vi "test_client_builder_configured.vi"() -> ()   [LabVIEW 2020, in "reqwest_tests.lvlib"]
uses:
  reqwest_tests.lvlib
  <vilib>/addons/_JKI Toolkits/Caraya/classes/Assert/Assert.lvclass
  <vilib>/addons/_JKI Toolkits/Caraya/classes/Test/Test.lvclass
  ClientBuilder/ClientBuilder.lvclass
  Client/Client.lvclass
panel:
  in  "error in (no error)":errorcluster
  out "error out":errorcluster
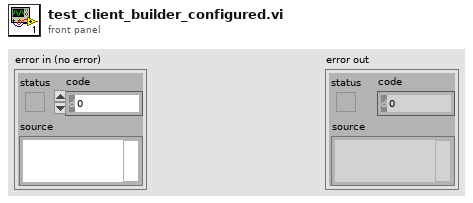
[diagram p1: front panel]
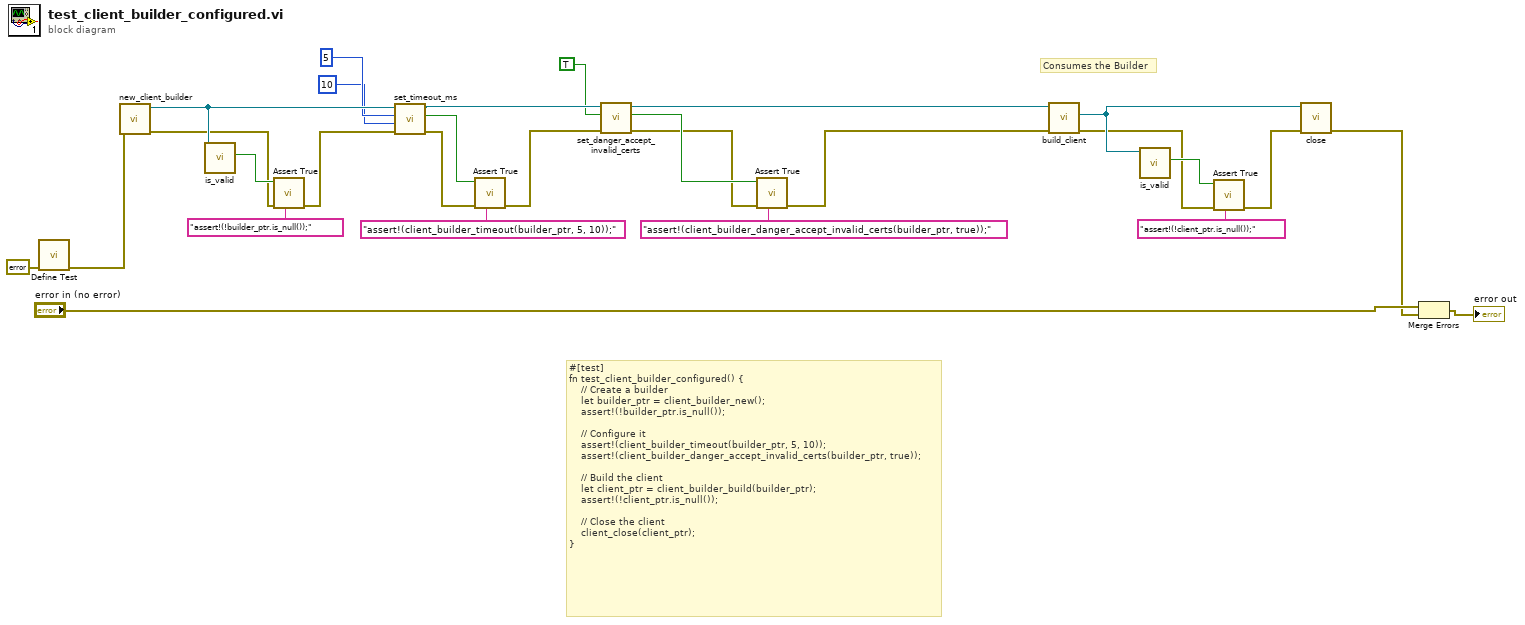
[diagram p0: block diagram]
diagram:
  # "Consumes the Builder"
  # "#[test]\nfn test_client_builder_configured() {\n    // Create a builder\n    let builder_ptr = client_builder_new();\n    assert!(!builder_ptr.is_null());\n\n    // Configure it\n    assert!(client_builder_timeout(builder_ptr, 5, 10));\n    assert!(client_builder_danger_accept_invalid_certs(builder_ptr, true));\n\n    // Build the client\n    let client_ptr = client_builder_build(builder_ptr);\n    assert!(!client_ptr.is_null());\n\n    // Close the client\n    client_close(client_ptr);\n}"
  n1 = call <vilib>:"Define Test.vi"("error in (no error)"=errorcluster {"status"=FALSE, "code"=0, "source"=""}) -> ("error out"=w9:errorcluster)  [unwired: 9 in, 1 out]
  n2 = call "new_client_builder.vi"("error in (no error)"=w9) -> ("error out"=w8:errorcluster, "Client out"=w23:refnum<class "ClientBuilder.lvclass">)  [unwired: 9 in]
  n3 = call "is_valid.vi"("Client in"=w23) -> ("valid-ref?"=w25:bool)  [unwired: 10 in]
  n4 = call <vilib>:"Assert True.vi"("Label"="assert!(!builder_ptr.is_null());", "error in (no error)"=w8, "True?"=w25) -> ("error out"=w7:errorcluster)  [unwired: 7 in, 1 out]
  n5 = call "set_timeout_ms.vi"("error in (no error)"=w7, "timeout_secs"=u64 10, 10:u64 5 ("connect_timeout_secs"), "ClientBuilder in"=w23) -> ("error out"=w6:errorcluster, "success"=w19:bool, "ClientBuilder out"=w18:refnum<class "ClientBuilder.lvclass">)  [unwired: 5 in]
  n6 = call <vilib>:"Assert True.vi"("Label"="assert!(client_builder_timeout(builder_ptr, 5, 10));", "error in (no error)"=w6, "True?"=w19) -> ("error out"=w5:errorcluster)  [unwired: 7 in, 1 out]
  n7 = call "set_danger_accept_invalid_certs.vi"("error in (no error)"=w5, "danger_accept_invalid_certs"=TRUE, "ClientBuilder in"=w18) -> ("error out"=w4:errorcluster, "success"=w15:bool, "ClientBuilder out"=w14:refnum<class "ClientBuilder.lvclass">)  [unwired: 6 in]
  n8 = call <vilib>:"Assert True.vi"("Label"="assert!(client_builder_danger_accept_invalid_certs(builder_ptr, true));", "error in (no error)"=w4, "True?"=w15) -> ("error out"=w3:errorcluster)  [unwired: 7 in, 1 out]
  n9 = call "build_client.vi"("error in (no error)"=w3, "ClientBuilder in"=w14) -> ("error out"=w2:errorcluster, "Client out"=w11:refnum<class "Client.lvclass">)  [unwired: 8 in]
  n10 = call "is_valid.vi"("Client in"=w11) -> ("valid-ref?"=w13:bool)  [unwired: 10 in]
  n11 = call <vilib>:"Assert True.vi"("Label"="assert!(!client_ptr.is_null());", "error in (no error)"=w2, "True?"=w13) -> ("error out"=w1:errorcluster)  [unwired: 7 in, 1 out]
  n12 = call "close.vi"("error in (no error)"=w1, "Client in"=w11) -> ("error out"=w10:errorcluster)  [unwired: 9 in]
  n13 = Merge Errors("error in (no error)", w10) -> (→"error out":errorcluster)
